vi "Configure Multi-Point [MP] Core.vi"(5 "sample interval (0.0 s)":dbl format="%.3f", 7 "sample trigger (Immediate)":i32(ring)=1 items=["Immediate"=1, "External"=2, "Software Trigger Function"=3, "Interval"=10, "PXI TRIG0 or VXI TTL0"=111, "PXI TRIG1 or VXI TTL1"=112, "PXI TRIG2 or VXI TTL2"=113, "PXI TRIG3 or VXI TTL3"=114, "PXI TRIG4 or VXI TTL4"=115, "PXI TRIG5 or VXI TTL5"=116, "PXI TRIG6 or VXI TTL6"=117, "PXI TRIG7 or VXI TTL7"=118, "ECL0"=119, "ECL1"=120, "PXI Star"=131, "RTSI 0"=140, "RTSI 1"=141, "RTSI 2"=142, "RTSI 3"=143, "RTSI 4"=144, "RTSI 5"=145, "RTSI 6"=146], 8 "error in (no error)":errorcluster, 9 "sample count (1)":i32=1, 10 "trigger count (1)":i32=1, 11 "IVI_DMM in":refnum<class "IVI_DMM.lvclass">) -> (0 "error out":errorcluster, 3 "IVI_DMM out":refnum<class "IVI_DMM.lvclass">)   [LabVIEW 2013, in "IVI_DMM.lvlib" / "IVI_DMM.lvclass"]
doc: "This VI configures the properties that affect multi-point measurements. These properties are the trigger count, sample count, sample trigger and sample interval.\n\nNote:\n\n(1) This VI is part of the IviDmmMultiPoint [MP] extension group."
uses:
  IVI_DMM.lvclass
  IVI_DMM.lvclass/IVI_DMM.ctl
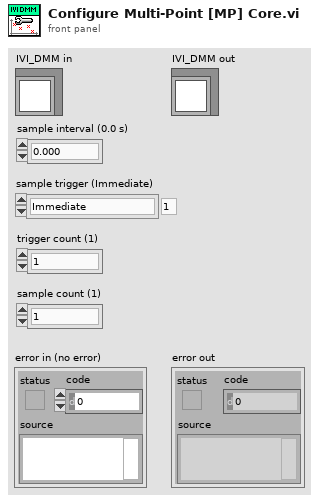
[diagram p1: front panel]
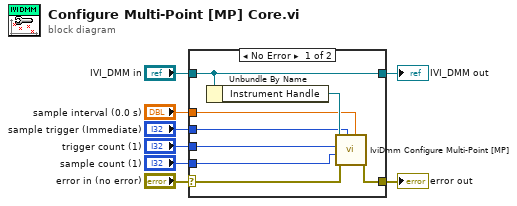
[diagram p0: block diagram]
diagram:
  n1 = case shown="No Error" "error in (no error)" {
    selector: "error in (no error)" -> [w13 w18]
    tunnel: [w15 w18] -> w7
    tunnel: [w16 w17] -> w5
    tunnel: "IVI_DMM in" -> [w16 w17]
    tunnel: "trigger count (1)" -> [w12 _]
    tunnel: "sample count (1)" -> [w11 _]
    tunnel: "sample trigger (Immediate)" -> [w10 _]
    tunnel: "sample interval (0.0 s)" -> [w9 _]
    frame No Error {
      n2 = Unbundle By Name(w16) -> ("Instrument Handle"=w14:refnum<k15>)
      n3 = call <vilib>:"IviDmm Configure Multi-Point [MP].vi"("sample interval (0.0 s)"=w9, "sample trigger (Immediate)"=w10, "error in (no error)"=w13, "sample count (1)"=w11, "trigger count (1)"=w12, "instrument handle"=w14) -> ("error out"=w15:errorcluster)  [unwired: 4 in, 1 out]
    }
    frame Error {
    }
  }
  "error out" <- w7
  "IVI_DMM out" <- w5
